vi "test - Find Disable Structure invalid.vi"(8 "error in (no error)":errorcluster, 11 "TestCase in":refnum<class "Find Disable Structure.lvclass">) -> (0 "error out":errorcluster, 3 "TestCase out":refnum<class "Find Disable Structure.lvclass">)   [LabVIEW 2018, in "Find Disable Structure.lvclass"]
uses:
  Find Disable Structure.lvclass
  <vilib>/addons/_JKI Toolkits/VI Tester/TestCase.llb/TestCase.lvclass
  C:/Program Files (x86)/National Instruments/LabVIEW 2018/vi.lib/addons/_JKI Toolkits/VI Tester/TestCase.llb/TestCase.lvclass
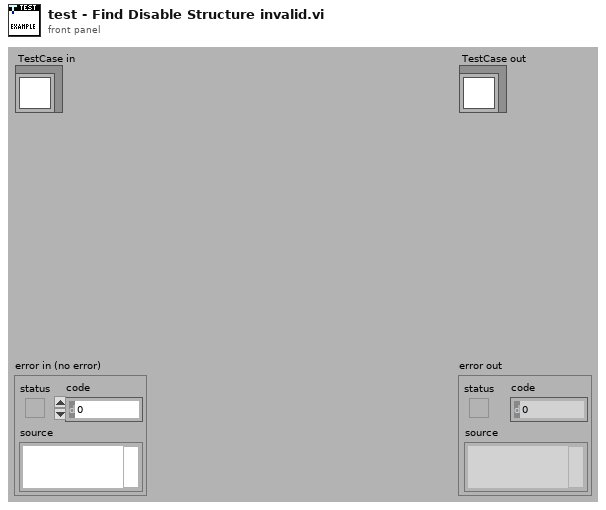
[diagram p1: front panel]
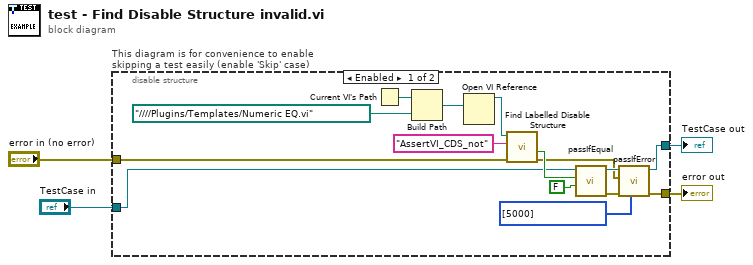
[diagram p0: block diagram]
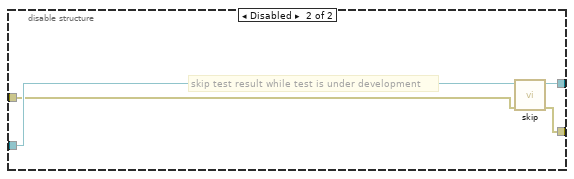
[diagram p2: hidden frame]
diagram:
  n1 = disable-structure "This diagram is for convenience to enable skipping a test easily (enable 'Skip' case)" shown="Enabled" {
    disable-tunnel: "TestCase in" -> [w14 w23]
    disable-tunnel: [w11 w21] -> w1
    disable-tunnel: [w13 w22] -> w3
    disable-tunnel: "error in (no error)" -> [w19 w20]
    frame Enabled {
      n2 = Current VI's Path() -> (path=w6:path)
      n3 = Build Path(base path=w6, name or relative path=path "../../../../Plugins/Templates/Numeric EQ.vi" ("vi path")) -> (appended path=w5:path)
      n4 = Open VI Reference(vi path=w5) -> (vi reference=w18:refnum<vi>)  [unwired: 5 in, 1 out]
      n5 = call "Find Labelled Disable Structure.vi"("error in (no error)"=w19, "Label"="AssertVI_CDS_not", "VI in"=w18) -> ("error out"=w9:errorcluster, "Found?"=w16:bool)  [unwired: 6 in, 1 out]
      n6 = call-dynamic "passIfEqual.vi"("y"=FALSE, "x"=w16, "TestCase in"=w14) -> ("error out"=w10:errorcluster, "TestCase out"=w12:refnum<class "Find Disable Structure.lvclass">)  [unwired: 7 in]
      n7 = call-dynamic "passIfError.vi"("passing error codes (default = any error code)"=i32[] [5000], "error in (no error)"=w10, "error"=w9, "TestCase in"=w12) -> ("error out"=w13:errorcluster, "TestCase out"=w11:refnum<class "Find Disable Structure.lvclass">)  [unwired: 6 in]
    }
    frame Disabled {
      # "skip test result while test is under development"
      n8 = call <vilib>:"skip.vi"("error in (no error)"=w20, "TestCase in"=w23) -> ("error out"=w22:errorcluster, "TestCase out"=w21:refnum<class "Find Disable Structure.lvclass">)  [unwired: 8 in]
    }
  }
  "error out" <- w3
  "TestCase out" <- w1
